vi "PID 1.vi"(8 "error in (no error)":errorcluster, 11 "State in":T1={"State"=enum."Idle", "Start Time"=timestamp(0 s since 1904-01-01), "Configuration"={"Cycle Period"=0.0, "PID 2 Parameters"={"Input Device"=enum."4-20mA", "Output Device"=enum."Default", "Setpoint"=0.0, "PID gains"={"proportional gain (Kc)"=0.0, "integral time (Ti, min)"=0.0, "derivative time (Td, min)"=100.0}, "output range"={"output low"=0.0, "output high"=1.0}}, "Manual Entry"=0.0, "Auto?"=TRUE, "4-20mA Input Settings"={"Input Channel "=0}, "4-20mA Out Settings"={"Output DAQ Task"=""}, "Input Channel Tag Name "=""}, "Current Time"=timestamp(0 s since 1904-01-01), "PID 1 Parameters"={"Setpoint"=0.0, "PID gains"={"proportional gain (Kc)"=1.0, "integral time (Ti, min)"=0.01, "derivative time (Td, min)"=0.0}}, "First Iteration"=FALSE, "Data"={"4-20mA Input"=0.0, "PID 2 Process Variable"=0.0, "PID 2 Output"=0.0, "4-20mA Output"=0.0}, "Process Name"="", "Pump On?"=enum."Off", "Input Error"=FALSE, "Output Error"=FALSE, "Log Started"=FALSE, "Current Setpoint"=0.0} {"Configuration"."PID 2 Parameters"."output range"."output low" format="%.2f"; "Configuration"."PID 2 Parameters"."output range"."output high" min=0.0 max=100.0 format="%.2f"; "Configuration"."PID 2 Parameters"."PID gains"."derivative time (Td, min)" format="%.3f"; "Configuration"."PID 2 Parameters"."PID gains"."integral time (Ti, min)" format="%.3f"; "Configuration"."PID 2 Parameters"."PID gains"."proportional gain (Kc)" format="%.3f"; "PID 1 Parameters"."PID gains"."derivative time (Td, min)" format="%.3f"; "PID 1 Parameters"."PID gains"."integral time (Ti, min)" format="%.3f"; "PID 1 Parameters"."PID gains"."proportional gain (Kc)" format="%.3f"}) -> (0 "error out":errorcluster, 3 "State out":T1={"State"=enum."Idle", "Start Time"=timestamp(0 s since 1904-01-01), "Configuration"={"Cycle Period"=0.0, "PID 2 Parameters"={"Input Device"=enum."4-20mA", "Output Device"=enum."Default", "Setpoint"=0.0, "PID gains"={"proportional gain (Kc)"=0.0, "integral time (Ti, min)"=0.0, "derivative time (Td, min)"=100.0}, "output range"={"output low"=0.0, "output high"=1.0}}, "Manual Entry"=0.0, "Auto?"=TRUE, "4-20mA Input Settings"={"Input Channel "=0}, "4-20mA Out Settings"={"Output DAQ Task"=""}, "Input Channel Tag Name "=""}, "Current Time"=timestamp(0 s since 1904-01-01), "PID 1 Parameters"={"Setpoint"=0.0, "PID gains"={"proportional gain (Kc)"=1.0, "integral time (Ti, min)"=0.01, "derivative time (Td, min)"=0.0}}, "First Iteration"=FALSE, "Data"={"4-20mA Input"=0.0, "PID 2 Process Variable"=0.0, "PID 2 Output"=0.0, "4-20mA Output"=0.0}, "Process Name"="", "Pump On?"=enum."Off", "Input Error"=FALSE, "Output Error"=FALSE, "Log Started"=FALSE, "Current Setpoint"=0.0} {"Configuration"."PID 2 Parameters"."output range"."output low" format="%.2f"; "Configuration"."PID 2 Parameters"."output range"."output high" min=0.0 max=100.0 format="%.2f"; "Configuration"."PID 2 Parameters"."PID gains"."derivative time (Td, min)" format="%.3f"; "Configuration"."PID 2 Parameters"."PID gains"."integral time (Ti, min)" format="%.3f"; "Configuration"."PID 2 Parameters"."PID gains"."proportional gain (Kc)" format="%.3f"; "PID 1 Parameters"."PID gains"."derivative time (Td, min)" format="%.3f"; "PID 1 Parameters"."PID gains"."integral time (Ti, min)" format="%.3f"; "PID 1 Parameters"."PID gains"."proportional gain (Kc)" format="%.3f"})   [LabVIEW 2018, in "4-20mA Module.lvlib" / "4-20mA Module Engine.lvlib"]
uses:
  4-20mA Module Engine.lvlib
  State Cluster.ctl
  State Enum.ctl
  Pressure Transmitter/Pressure Transmitter Device Settings.ctl
  Pressure Reg Module/Pressure Regulator Device Settings.ctl
  Measure Instrument/PID 1 Parameters Cluster.ctl
  <vilib>/addons/control/pid/NI_PID_pid.lvlib
  <vilib>/addons/control/pid/pid.llb/PID (DBL).vi
  Pressure Transmitter/Pressure Transmitter Library.lvlib
  Pressure Reg Module/Pressure Regulator Library.lvlib
panel:
  # "Instrument Settings"
  # "Instrument Settings"
  # "Instrument Settings"
  # "Instrument Settings"
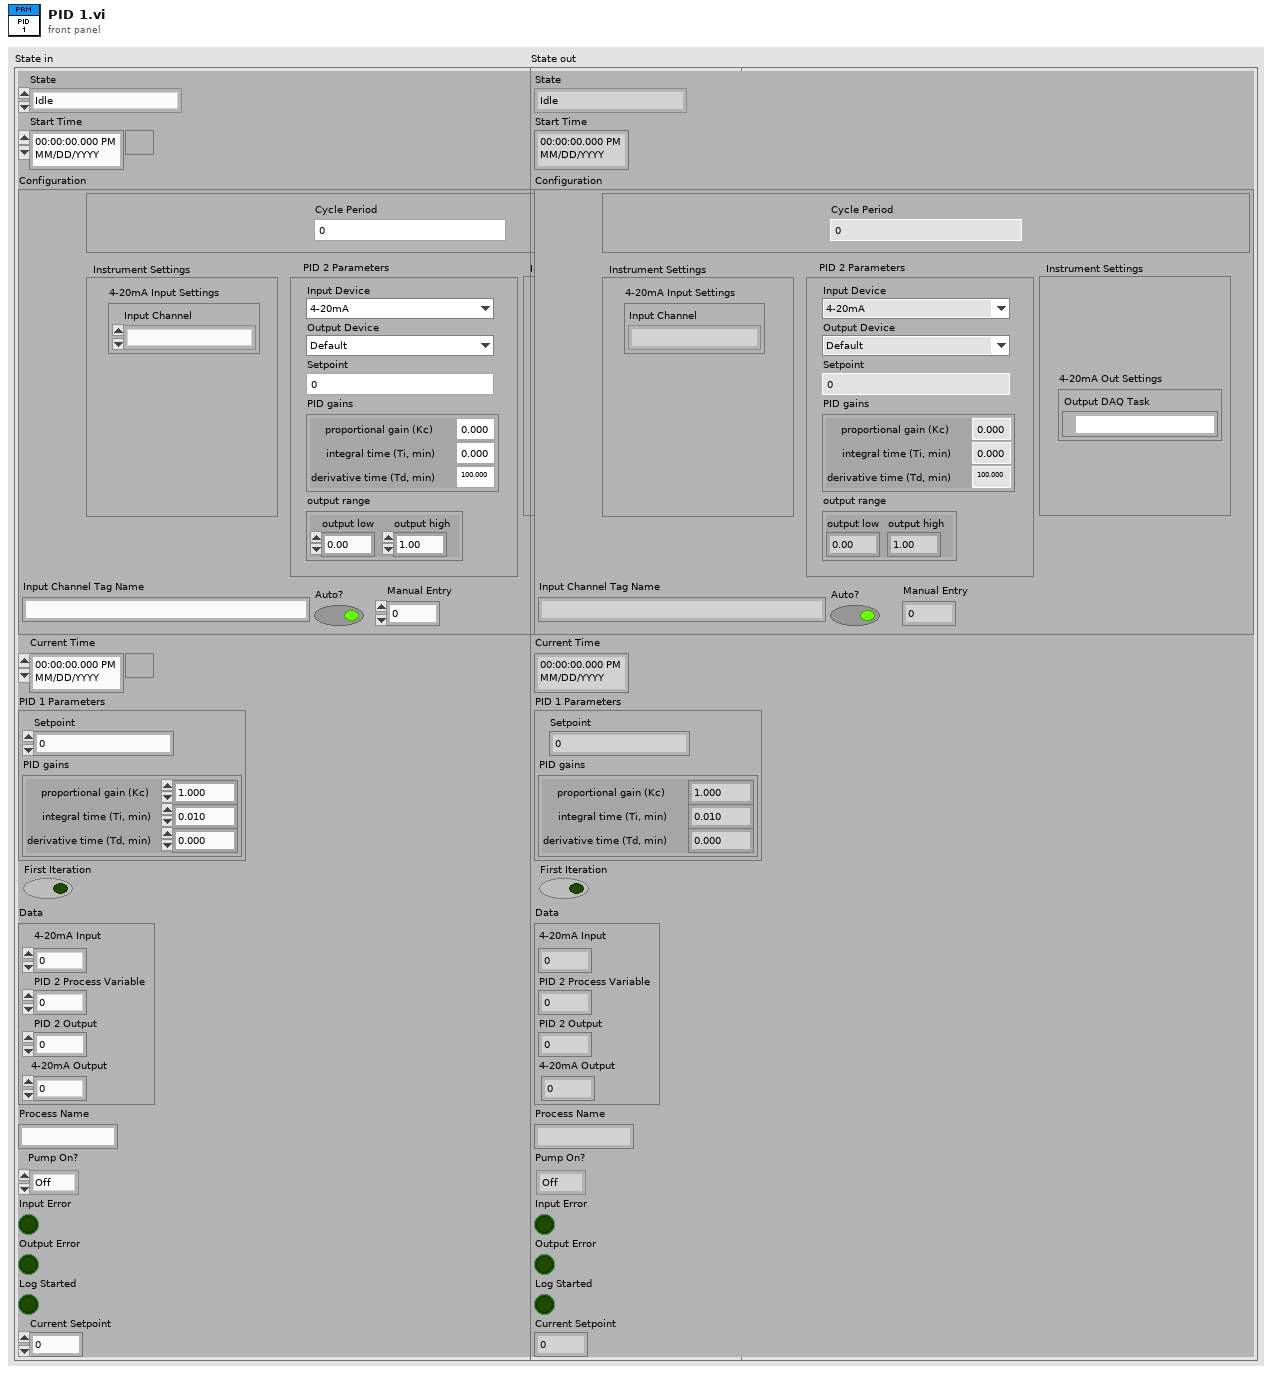
[diagram p1: front panel]
types:
  T1 = typedef "4-20mA Module.lvlib/4-20mA Module Engine.lvlib/State Cluster.ctl" = cluster{"State":T2, "Start Time":timestamp, "Configuration":cluster{"Cycle Period":dbl, "PID 2 Parameters":cluster{"Input Device":enum16{"Default", "4-20mA"}, "Output Device":enum16{"Default", "Equilibar Pressure Reg", "Flow Regulator"}, "Setpoint":dbl, "PID gains":cluster{"proportional gain (Kc)":dbl, "integral time (Ti, min)":dbl, "derivative time (Td, min)":dbl}, "output range":cluster{"output low":dbl, "output high":dbl}}, "Manual Entry":dbl, "Auto?":bool, "4-20mA Input Settings":T3, "4-20mA Out Settings":T4, "Input Channel Tag Name ":string}, "Current Time":timestamp, "PID 1 Parameters":T5, "First Iteration":bool, "Data":cluster{"4-20mA Input":dbl, "PID 2 Process Variable":dbl, "PID 2 Output":dbl, "4-20mA Output":dbl}, "Process Name":string, "Pump On?":enum16{"Off", "On", "Not Initialized"}, "Input Error":bool, "Output Error":bool, "Log Started":bool, "Current Setpoint":dbl}
  T2 = typedef "4-20mA Module.lvlib/4-20mA Module Engine.lvlib/State Enum.ctl" = enum16{"Measuring", "Idle", "Paused"}
  T3 = typedef "Pressure Transmitter Library.lvlib/Pressure Transmitter Device Settings.ctl" = cluster{"Input Channel ":u16}
  T4 = typedef "Pressure Regulator Library.lvlib/Pressure Regulator Device Settings.ctl" = cluster{"Output DAQ Task":refnum<k21>}
  T5 = typedef "PID 1 Parameters Cluster.ctl" = cluster{"Setpoint":dbl, "PID gains":cluster{"proportional gain (Kc)":dbl, "integral time (Ti, min)":dbl, "derivative time (Td, min)":dbl}}
  T6 = cluster{"proportional gain (Kc)":dbl, "integral time (Ti, min)":dbl, "derivative time (Td, min)":dbl}
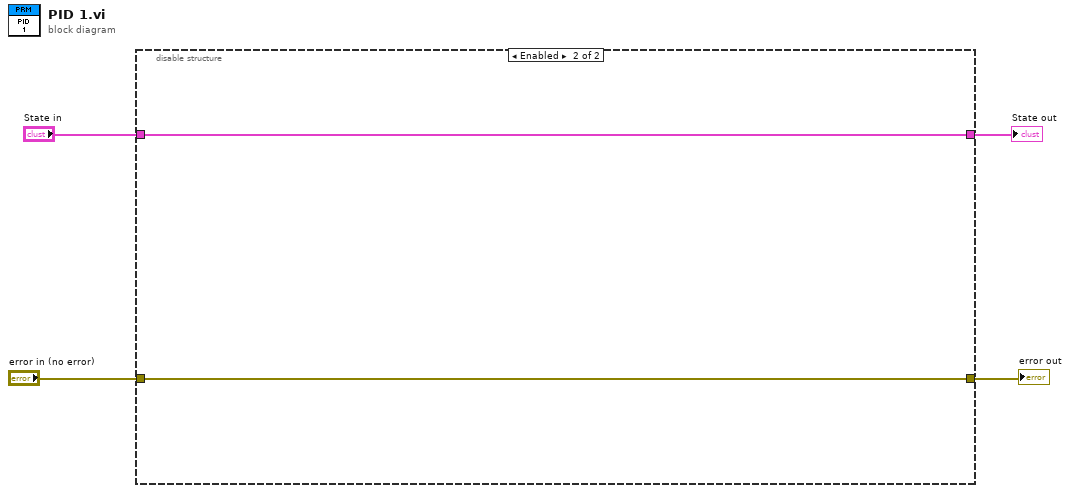
[diagram p0: block diagram]
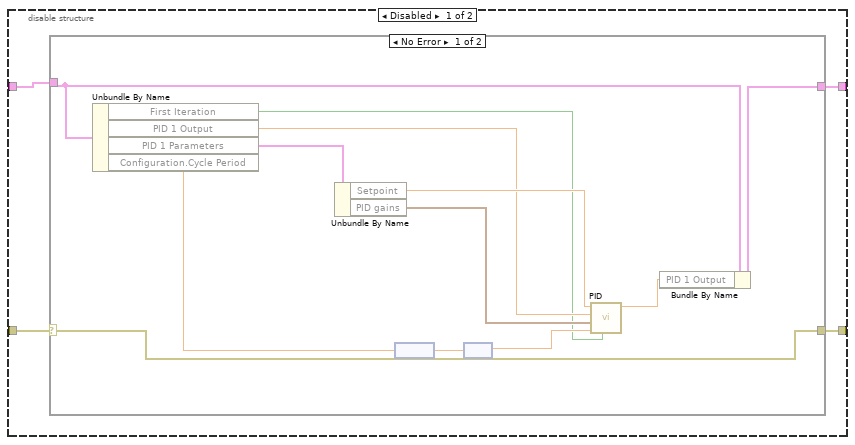
[diagram p2: hidden frame]
diagram:
  n1 = disable-structure shown="Enabled" {
    disable-tunnel: "error in (no error)" -> [w8 w23]
    disable-tunnel: [w7 w23] -> w3
    disable-tunnel: "State in" -> [w6 w24]
    disable-tunnel: [w5 w24] -> w1
    frame Disabled {
      n2 = case shown="No Error" w8 {
        selector: w8 -> [w16 w22]
        tunnel: [w16 w22] -> w7
        tunnel: w6 -> [w13 w21]
        tunnel: [w14 w21] -> w5
        frame No Error {
          n3 = Unbundle By Name(w13) -> ("First Iteration"=w9:bool, "PID 1 Output"=w11:dbl, "PID 1 Parameters"=w12:T5, "Configuration.Cycle Period"=w10:dbl)
          n4 = Unbundle By Name(w12) -> ("Setpoint"=w20:dbl, "PID gains"=w19:T6)
          n5 = node(w10) -> (w18:dbl[unit])
          n6 = node(w18) -> (w17:dbl)
          n7 = call-poly <vilib>:"PID.vi"("reinitialize? (F)"=w9, "dt (s)"=w17, "PID gains"=w19, "process variable"=w11, "setpoint"=w20) -> ("output"=w15:dbl)  [unwired: 5 in, 1 out]
          n8 = Bundle By Name(cluster=w13, "PID 1 Output"=w15) -> (w14:T1)
        }
        frame Error {
        }
      }
    }
    frame Enabled {
    }
  }
  "error out" <- w3
  "State out" <- w1
